vi "Handle Error.vi"(8 "error in (no error)":errorcluster, 11 "Actor Tests in":refnum<class "Actor Tests.lvclass">) -> (0 "error out":errorcluster, 2 "stop actor?":bool=TRUE, 3 "Actor Tests out":refnum<class "Actor Tests.lvclass">)   [LabVIEW 2020, in "Actor Tests.lvlib" / "Actor Tests.lvclass"]
doc: "(<B>Filename</B>: Actor Framework.lvlib:Actor.lvclass:Handle Error.vi)\n\nDefines how the actor handles an error that occurred while processing a message. By default, this method does nothing except stop the actor."
uses:
  Actor Tests.lvclass
  <vilib>/ActorFramework/Actor/Actor.lvclass
  Actor Tests.lvclass/Actor Tests.ctl
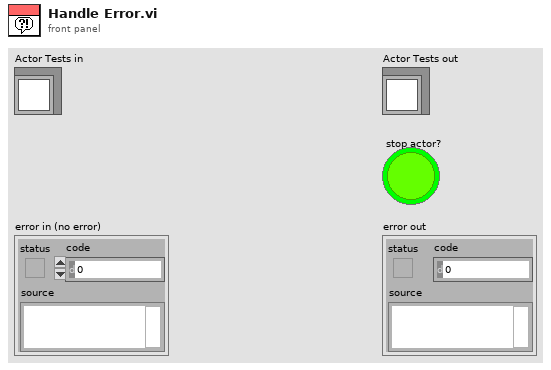
[diagram p1: front panel]
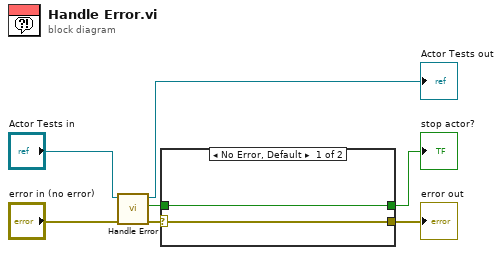
[diagram p0: block diagram]
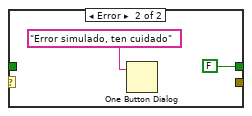
[diagram p2: hidden frame]
diagram:
  n1 = call-parent "Handle Error.vi"("error in (no error)"="error in (no error)", "Actor in"="Actor Tests in") -> ("error out"=w4:errorcluster, "stop actor?"=w2:bool, "Actor out"=→"Actor Tests out":refnum<class "Actor Tests.lvclass">)  [unwired: 7 in]
  n2 = case shown="No Error, Default" w4 {
    selector: w4 -> [w9 _]
    tunnel: [w9 _] -> w3
    tunnel: w2 -> [w8 _]
    tunnel: [w8 FALSE ("stop actor?")] -> w1
    frame No Error {
    }
    frame Error {
      n3 = One Button Dialog(message="Error simulado, ten cuidado") -> ()  [unwired: 1 in, 1 out]
    }
  }
  "error out" <- w3
  "stop actor?" <- w1
